vi "HandleSrvs.vi"(8 "error in (no error)":errorcluster, 11 "S4GUI in":refnum<class "S4GUI.lvclass">) -> (0 "error out":errorcluster, 3 "S4GUI out":refnum<class "S4GUI.lvclass">)   [LabVIEW 2018, in "S4GUI.lvclass"]
uses:
  S4GUI.lvclass
  S4GUI.lvclass/S4GUI.ctl
  Instrument/Instrument.lvclass/Instrument.ctl
  Device/Optics/Opt_Selector/Opt_Selector.lvclass
  SyncBox/Sync Box.lvclass
  Acquisition/Acquisition.lvclass
  Instrument/Instrument.lvclass
  Channel/Channel.lvclass
  Trigger/Trigger.lvclass
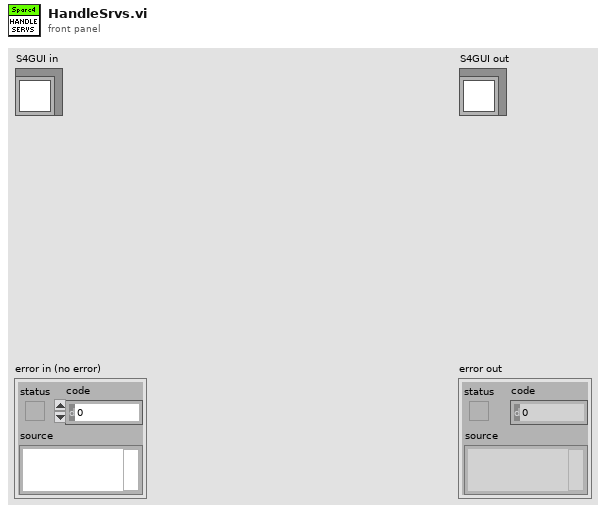
[diagram p1: front panel]
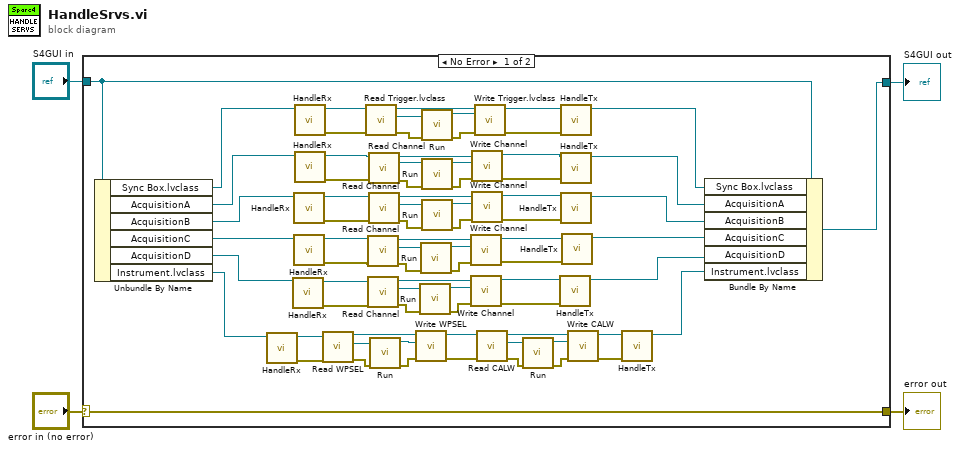
[diagram p0: block diagram]
diagram:
  n1 = case shown="No Error" "error in (no error)" {
    selector: "error in (no error)" -> [w80 w82]
    tunnel: [w80 w82] -> w3
    tunnel: [w77 w81] -> w1
    tunnel: "S4GUI in" -> [w78 w81]
    frame No Error {
      n2 = Unbundle By Name(w78) -> ("Sync Box.lvclass"=w44:refnum<class "Sync Box.lvclass">, "AcquisitionA"=w34:refnum<class "Acquisition.lvclass">, "AcquisitionB"=w32:refnum<class "Acquisition.lvclass">, "AcquisitionC"=w30:refnum<class "Acquisition.lvclass">, "AcquisitionD"=w23:refnum<class "Acquisition.lvclass">, "Instrument.lvclass"=w22:refnum<class "Instrument.lvclass">)
      n3 = call-dynamic "HandleRx.vi"("Server in"=w22) -> ("error out"=w20:errorcluster, "Server out"=w21:refnum<class "Instrument.lvclass">)  [unwired: 9 in]
      n4 = call-dynamic "HandleRx.vi"("Server in"=w23) -> ("error out"=w25:errorcluster, "Server out"=w24:refnum<class "Acquisition.lvclass">)  [unwired: 9 in]
      n5 = call-dynamic "HandleRx.vi"("Server in"=w32) -> ("error out"=w27:errorcluster, "Server out"=w31:refnum<class "Acquisition.lvclass">)  [unwired: 9 in]
      n6 = call-dynamic "HandleRx.vi"("Server in"=w30) -> ("error out"=w26:errorcluster, "Server out"=w29:refnum<class "Acquisition.lvclass">)  [unwired: 9 in]
      n7 = call-dynamic "HandleRx.vi"("Server in"=w44) -> ("error out"=w35:errorcluster, "Server out"=w43:refnum<class "Sync Box.lvclass">)  [unwired: 9 in]
      n8 = call-dynamic "HandleRx.vi"("Server in"=w34) -> ("error out"=w28:errorcluster, "Server out"=w33:refnum<class "Acquisition.lvclass">)  [unwired: 9 in]
      n9 = call "Read WPSEL.vi"("error in (no error)"=w20, "Instrument in"=w21) -> ("error out"=w53:errorcluster, "Opt_Selector.lvclass"=w55:refnum<class "Opt_Selector.lvclass">, "Instrument out"=w56:refnum<class "Instrument.lvclass">)  [unwired: 7 in]
      n10 = call-dynamic "Read Trigger.lvclass.vi"("error in (no error)"=w35, "Sync Box in"=w43) -> ("error out"=w38:errorcluster, "Trigger.lvclass"=w40:refnum<class "Trigger.lvclass">, "Sync Box out"=w79:refnum<class "Sync Box.lvclass">)  [unwired: 7 in]
      n11 = call-dynamic "Read Channel.vi"("error in (no error)"=w26, "Acquisition in"=w29) -> ("error out"=w69:errorcluster, "Channel.lvclass"=w61:refnum<class "Channel.lvclass">, "Acquisition out"=w62:refnum<class "Acquisition.lvclass">)  [unwired: 7 in]
      n12 = call-dynamic "Read Channel.vi"("error in (no error)"=w25, "Acquisition in"=w24) -> ("error out"=w67:errorcluster, "Channel.lvclass"=w58:refnum<class "Channel.lvclass">, "Acquisition out"=w59:refnum<class "Acquisition.lvclass">)  [unwired: 7 in]
      n13 = call-dynamic "Read Channel.vi"("error in (no error)"=w28, "Acquisition in"=w33) -> ("error out"=w73:errorcluster, "Channel.lvclass"=w76:refnum<class "Channel.lvclass">, "Acquisition out"=w74:refnum<class "Acquisition.lvclass">)  [unwired: 7 in]
      n14 = call-dynamic "Read Channel.vi"("error in (no error)"=w27, "Acquisition in"=w31) -> ("error out"=w71:errorcluster, "Channel.lvclass"=w65:refnum<class "Channel.lvclass">, "Acquisition out"=w63:refnum<class "Acquisition.lvclass">)  [unwired: 7 in]
      n15 = call-dynamic "Run.vi"("error in (no error)"=w53, "Opctics in"=w55) -> ("error out"=w52:errorcluster, "Opt_Selector out"=w54:refnum<class "Opt_Selector.lvclass">)  [unwired: 8 in]
      n16 = call "Write WPSEL.vi"("error in (no error)"=w52, "Opt_Selector.lvclass"=w54, "Instrument in"=w56) -> ("error out"=w45:errorcluster, "Instrument out"=w49:refnum<class "Instrument.lvclass">)  [unwired: 7 in]
      n17 = call-dynamic "Run.vi"("error in (no error)"=w67, "Channel in"=w58) -> ("error out"=w66:errorcluster, "Channel out"=w57:refnum<class "Channel.lvclass">)  [unwired: 8 in]
      n18 = call-dynamic "Run.vi"("error in (no error)"=w69, "Channel in"=w61) -> ("error out"=w68:errorcluster, "Channel out"=w60:refnum<class "Channel.lvclass">)  [unwired: 8 in]
      n19 = call-dynamic "Run.vi"("error in (no error)"=w38, "Trigger in"=w40) -> ("error out"=w37:errorcluster, "Trigger out"=w39:refnum<class "Trigger.lvclass">)  [unwired: 8 in]
      n20 = call-dynamic "Run.vi"("error in (no error)"=w73, "Channel in"=w76) -> ("error out"=w72:errorcluster, "Channel out"=w75:refnum<class "Channel.lvclass">)  [unwired: 8 in]
      n21 = call-dynamic "Run.vi"("error in (no error)"=w71, "Channel in"=w65) -> ("error out"=w70:errorcluster, "Channel out"=w64:refnum<class "Channel.lvclass">)  [unwired: 8 in]
      n22 = call-dynamic "Write Channel.vi"("error in (no error)"=w68, "Channel.lvclass"=w60, "Acquisition in"=w62) -> ("error out"=w11:errorcluster, "Acquisition out"=w13:refnum<class "Acquisition.lvclass">)  [unwired: 7 in]
      n23 = call-dynamic "Write Channel.vi"("error in (no error)"=w66, "Channel.lvclass"=w57, "Acquisition in"=w59) -> ("error out"=w9:errorcluster, "Acquisition out"=w10:refnum<class "Acquisition.lvclass">)  [unwired: 7 in]
      n24 = call-dynamic "Write Channel.vi"("error in (no error)"=w72, "Channel.lvclass"=w75, "Acquisition in"=w74) -> ("error out"=w17:errorcluster, "Acquisition out"=w19:refnum<class "Acquisition.lvclass">)  [unwired: 7 in]
      n25 = call-dynamic "Write Channel.vi"("error in (no error)"=w70, "Channel.lvclass"=w64, "Acquisition in"=w63) -> ("error out"=w14:errorcluster, "Acquisition out"=w16:refnum<class "Acquisition.lvclass">)  [unwired: 7 in]
      n26 = call-dynamic "Write Trigger.lvclass.vi"("error in (no error)"=w37, "Trigger.lvclass"=w39, "Sync Box in"=w79) -> ("error out"=w36:errorcluster, "Sync Box out"=w42:refnum<class "Sync Box.lvclass">)  [unwired: 7 in]
      n27 = call "Read CALW.vi"("error in (no error)"=w45, "Instrument in"=w49) -> ("error out"=w51:errorcluster, "Opt_Selector.lvclass"=w47:refnum<class "Opt_Selector.lvclass">, "Instrument out"=w48:refnum<class "Instrument.lvclass">)  [unwired: 7 in]
      n28 = call-dynamic "Run.vi"("error in (no error)"=w51, "Opctics in"=w47) -> ("error out"=w50:errorcluster, "Opt_Selector out"=w46:refnum<class "Opt_Selector.lvclass">)  [unwired: 8 in]
      n29 = call-dynamic "HandleTx.vi"("error in (no error)"=w9, "Server in"=w10) -> ("Server out"=w8:refnum<class "Acquisition.lvclass">)  [unwired: 8 in, 1 out]
      n30 = call-dynamic "HandleTx.vi"("error in (no error)"=w36, "Server in"=w42) -> ("Server out"=w41:refnum<class "Sync Box.lvclass">)  [unwired: 8 in, 1 out]
      n31 = call-dynamic "HandleTx.vi"("error in (no error)"=w17, "Server in"=w19) -> ("Server out"=w18:refnum<class "Acquisition.lvclass">)  [unwired: 8 in, 1 out]
      n32 = call-dynamic "HandleTx.vi"("error in (no error)"=w14, "Server in"=w16) -> ("Server out"=w15:refnum<class "Acquisition.lvclass">)  [unwired: 8 in, 1 out]
      n33 = call-dynamic "HandleTx.vi"("error in (no error)"=w11, "Server in"=w13) -> ("Server out"=w12:refnum<class "Acquisition.lvclass">)  [unwired: 8 in, 1 out]
      n34 = call "Write CALW.vi"("error in (no error)"=w50, "Opt_Selector.lvclass"=w46, "Instrument in"=w48) -> ("error out"=w5:errorcluster, "Instrument out"=w7:refnum<class "Instrument.lvclass">)  [unwired: 7 in]
      n35 = call-dynamic "HandleTx.vi"("error in (no error)"=w5, "Server in"=w7) -> ("Server out"=w6:refnum<class "Instrument.lvclass">)  [unwired: 8 in, 1 out]
      n36 = Bundle By Name(cluster=w78, "Sync Box.lvclass"=w41, "AcquisitionA"=w18, "AcquisitionB"=w15, "AcquisitionC"=w12, "AcquisitionD"=w8, "Instrument.lvclass"=w6) -> (w77:refnum<class "S4GUI.lvclass">)
    }
    frame Error {
    }
  }
  "error out" <- w3
  "S4GUI out" <- w1
